vi "Part 5 Array Max & Min & Reshape Array.vi"() -> ()   [LabVIEW 2020]
panel:
  out "output array":dbl[][](array[numeric])
  out "min value":dbl
  out "max value":dbl
  in  "array":dbl[](array[numeric])
  # "Array Max & Min & Reshape Array"
  # "Array Max & Min"
  # "0       1          2"
  # "Reshape Array"
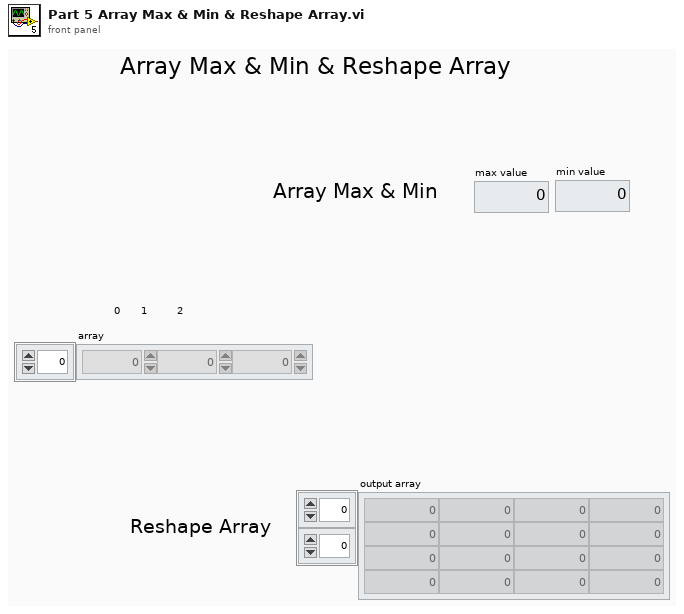
[diagram p1: front panel]
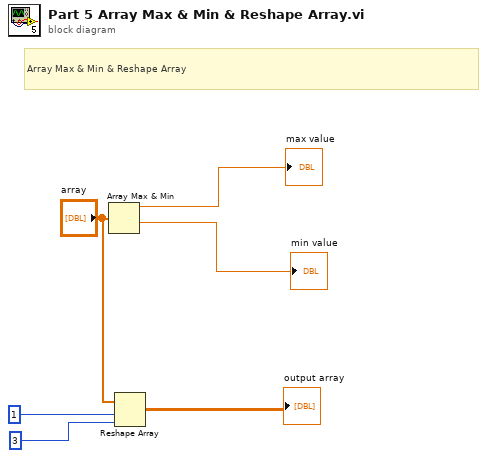
[diagram p0: block diagram]
diagram:
  # "Array Max & Min & Reshape Array"
  n1 = Array Max & Min(array="array") -> (max value=→"max value":dbl, min value=→"min value":dbl)  [unwired: 2 out]
  n2 = Reshape Array "Reshape Array"("array", 1 ("dimension size"), 3 ("dimension size")) -> (→"output array":dbl[][])
